vi "DAQ.Create AO Tasks.vi"(8 "error in (no error)":errorcluster, 11 "Instrument.DAQ":refnum<class "Instrument.DAQ.lvclass">) -> (0 "error out":errorcluster, 3 "Instrument.DAQ":refnum<class "Instrument.DAQ.lvclass">)   [LabVIEW 2019, in "Instrument.DAQ.lvclass"]
uses:
  Instrument.DAQ.lvclass
  Instrument.DAQ.lvclass/Instrument.DAQ.ctl
  <vilib>/DAQmx/create/channels.llb/DAQmx Create Channel (AO-Voltage-Basic).vi
  <resource>/objmgr/daqmx.rc
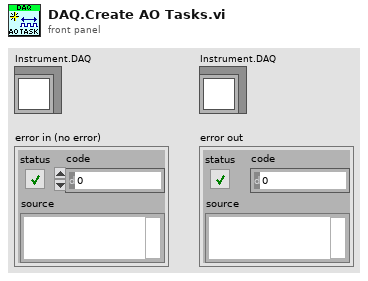
[diagram p1: front panel]
types:
  T1 = typedef "Instrument.DAQ.lvclass/DAQ.Config.AO--Cluster--Array.ctl" = T2[]
  T2 = typedef "Instrument.DAQ.lvclass/DAQ.Config.AO--Cluster.ctl" = cluster{"Channels":tag, "Range":T3, "output terminal configuration":i32, "Type":T4}
  T3 = typedef "Instrument.DAQ.lvclass/DAQ.Config.AO.Range--enum.ctl" = enum16{"±0.1", "±1.0", "±10.0"}
  T4 = typedef "Instrument.DAQ.lvclass/DAQ.Type--enum.ctl" = enum16{"None", "USB 4431", "PXI 446x"}
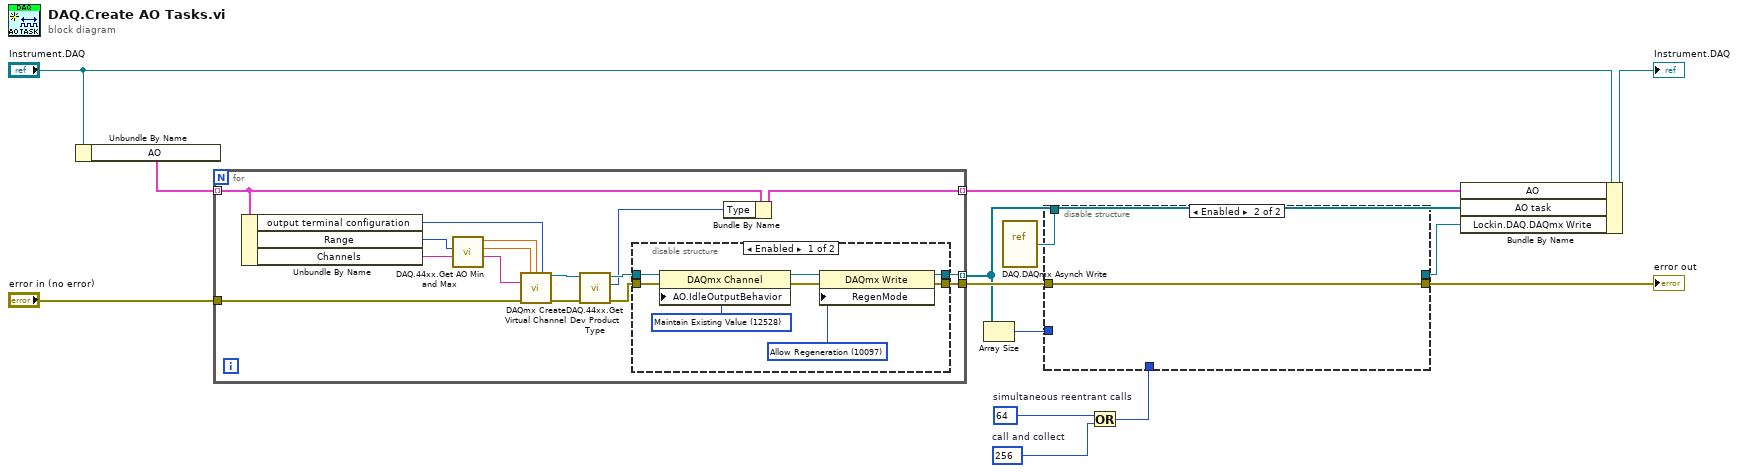
[diagram p0: block diagram]
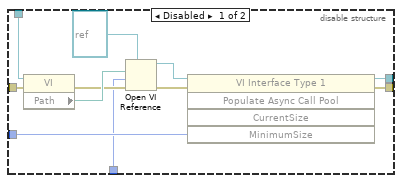
[diagram p3: hidden frame]
diagram:
  w5 = 64  # simultaneous reentrant calls
  w6 = 256  # call and collect
  n1 = Unbundle By Name("Instrument.DAQ") -> ("AO"=w3:T1)
  n2 = for {
    tunnel: "error in (no error)" -> [w30]
    tunnel: [w22] -> w9
    tunnel: w3 -> [w21] mode=indexing
    tunnel: [w23] -> w2 mode=indexing
    tunnel: [w24] -> w7 mode=indexing
    n3 = Unbundle By Name(w21) -> ("output terminal configuration"=w26:i32, "Range"=w25:T3, "Channels"=w27:tag)
    n4 = call "DAQ.44xx.Get AO Min and Max.vi"("AO.channels"=w27, "AO.Range"=w25) -> ("AO.channels out"=w20:tag, "AO.max"=w29:dbl, "AO.min"=w28:dbl)  [unwired: 7 in]
    n5 = call-poly <vilib>:"DAQmx Create Virtual Channel.vi"("maximum value"=w29, "minimum value"=w28, "output terminal configuration"=w26, "physical channels"=w20, "error in"=w30) -> ("task out"=w19:refnum<k21>, "error out"=w16:errorcluster)  [unwired: 9 in]
    n6 = call "DAQ.44xx.Get Dev Product Type.vi"("error in (no error)"=w16, "Refnum in"=w19) -> ("error out"=w18:errorcluster, "DAQ Type"=w15:T4, "Refnum out"=w17:refnum<k21>)  [unwired: 6 in, 1 out]
    n7 = disable-structure shown="Enabled" {
      disable-tunnel: w17 -> [w38 w40]
      disable-tunnel: [w35 w40] -> w24
      disable-tunnel: w18 -> [w34 w39]
      disable-tunnel: [w31 w39] -> w22
      frame Enabled {
        w32 = 10097 items=["Allow Regeneration"=10097, "Do Not Allow Regeneration"=10158] ("RegenMode")
        w33 = 12528 items=["Zero Volts"=12526, "High-Impedance"=12527, "Maintain Existing Value"=12528] ("AO.IdleOutputBehavior")
        n8 = property class="DAQmx Channel"(reference=w38, error in=w34, "AO.IdleOutputBehavior"=w33) -> (reference out=w37:refnum<k21>, error out=w36:errorcluster)
        n9 = property class="DAQmx Write"(reference=w37, error in=w36, "RegenMode"=w32) -> (reference out=w35:refnum<k21>, error out=w31:errorcluster)
      }
      frame Disabled {
      }
    }
    n10 = Bundle By Name(cluster=w21, "Type"=w15) -> (w23:T2)
  }
  n11 = Array Size(array=w7) -> (size(s)=w10:i32)
  n12 = vi-ref "DAQ.DAQmx Asynch Write.vi"() -> (w11:refnum<vi>)
  n13 = Or(x=w5, y=w6) -> (x .or. y?=w4:i32)
  n14 = disable-structure shown="Enabled" {
    disable-tunnel: w11 -> [w51 _]
    disable-tunnel: w10 -> [w45 _]
    disable-tunnel: w9 -> [w44 w52]
    disable-tunnel: [w43 w52] -> w8
    disable-tunnel: [w42 _] -> w1
    disable-tunnel: w4 -> [w41 _]
    frame Disabled {
      n15 = property class="VI"(reference=w51, error in=w44) -> (error out=w49:errorcluster, "Path"=w50:path)  [unwired: 1 out]
      n16 = Open VI Reference(type specifier VI Refnum (for type only)=refnum<vi> refnum, vi path=w50, options=w41, error in (no error)=w49) -> (vi reference=w47:refnum<vi>, error out=w46:errorcluster)  [unwired: 2 in]
      n17 = invoke class="VI Interface Type 1" method="Populate Async Call Pool"(reference=w47, error in=w46, "MinimumSize"=w45) -> (reference out=w42:refnum<vi>, error out=w43:errorcluster)  [unwired: 2 in, 3 out]
    }
    frame Enabled {
    }
  }
  "error out" <- w8
  n18 = Bundle By Name(cluster="Instrument.DAQ", "AO"=w2, "AO task"=w7, "Lockin.DAQ.DAQmx Write"=w1) -> (→"Instrument.DAQ":refnum<class "Instrument.DAQ.lvclass">)
